vi "Close.vi"(8 "error in (no error)":errorcluster, 11 "Ini File in":refnum<class "Ini File.lvclass">) -> (0 "error out":errorcluster)   [LabVIEW 2021, in "File Library.lvlib" / "Ini File.lvclass"]
uses:
  Ini File.lvclass
  Ini File.lvclass/Ini File.ctl
  <vilib>/Utility/config.llb/NI_LVConfig.lvlib
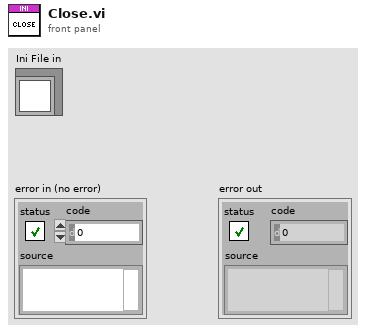
[diagram p1: front panel]
types:
  T1 = typedef "NI_LVConfig.lvlib/Config Data RefNum.ctl" = refnum<k1>
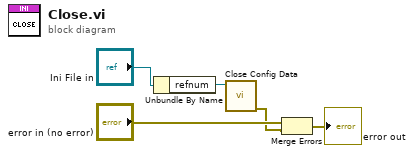
[diagram p0: block diagram]
diagram:
  n1 = Unbundle By Name("Ini File in") -> ("refnum"=w3:T1)
  n2 = call <vilib>:"Close Config Data.vi"("refnum"=w3) -> ("error out"=w1:errorcluster)  [unwired: 9 in, 1 out]
  n3 = Merge Errors("error in (no error)", w1) -> (→"error out":errorcluster)
